vi "Build Profile Header Commands.vi"(8 "error in":errorcluster, 9 "Profile Name":string, 10 "Profile Number":u32=1 min=1 step=1, 11 "F4T in":refnum<class "F4T.lvclass">) -> (0 "error out":errorcluster, 2 "Profile Header Commands":T1[](array[typedef]), 3 "F4T out":refnum<class "F4T.lvclass">)   [LabVIEW 2018, in "F4T.lvlib" / "F4T.lvclass"]
uses:
  F4T.lvclass
  Custom Controls/Command Data.ctl
  PPLs/Temp Chamber/Parent/Temp Chamber.lvlibp/Temp Chamber.lvclass
  PPLs/Temp Chamber/Parent/Configuration.lvlibp/Configuration.lvclass
  C:/Projects/LabVIEW/PPLs/Temp Chamber/Parent/Temp Chamber.lvlibp/Temp Chamber.lvclass
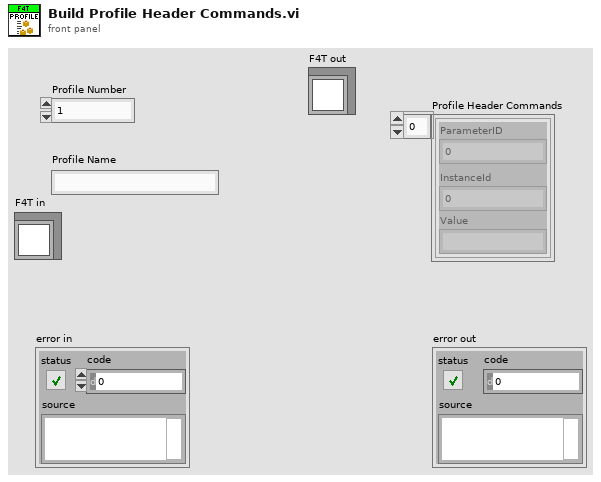
[diagram p1: front panel]
types:
  T1 = typedef "F4T.lvlib/F4T.lvclass/Command Data.ctl" = cluster{"ParameterID":u32, "InstanceId":u32, "Value":string}
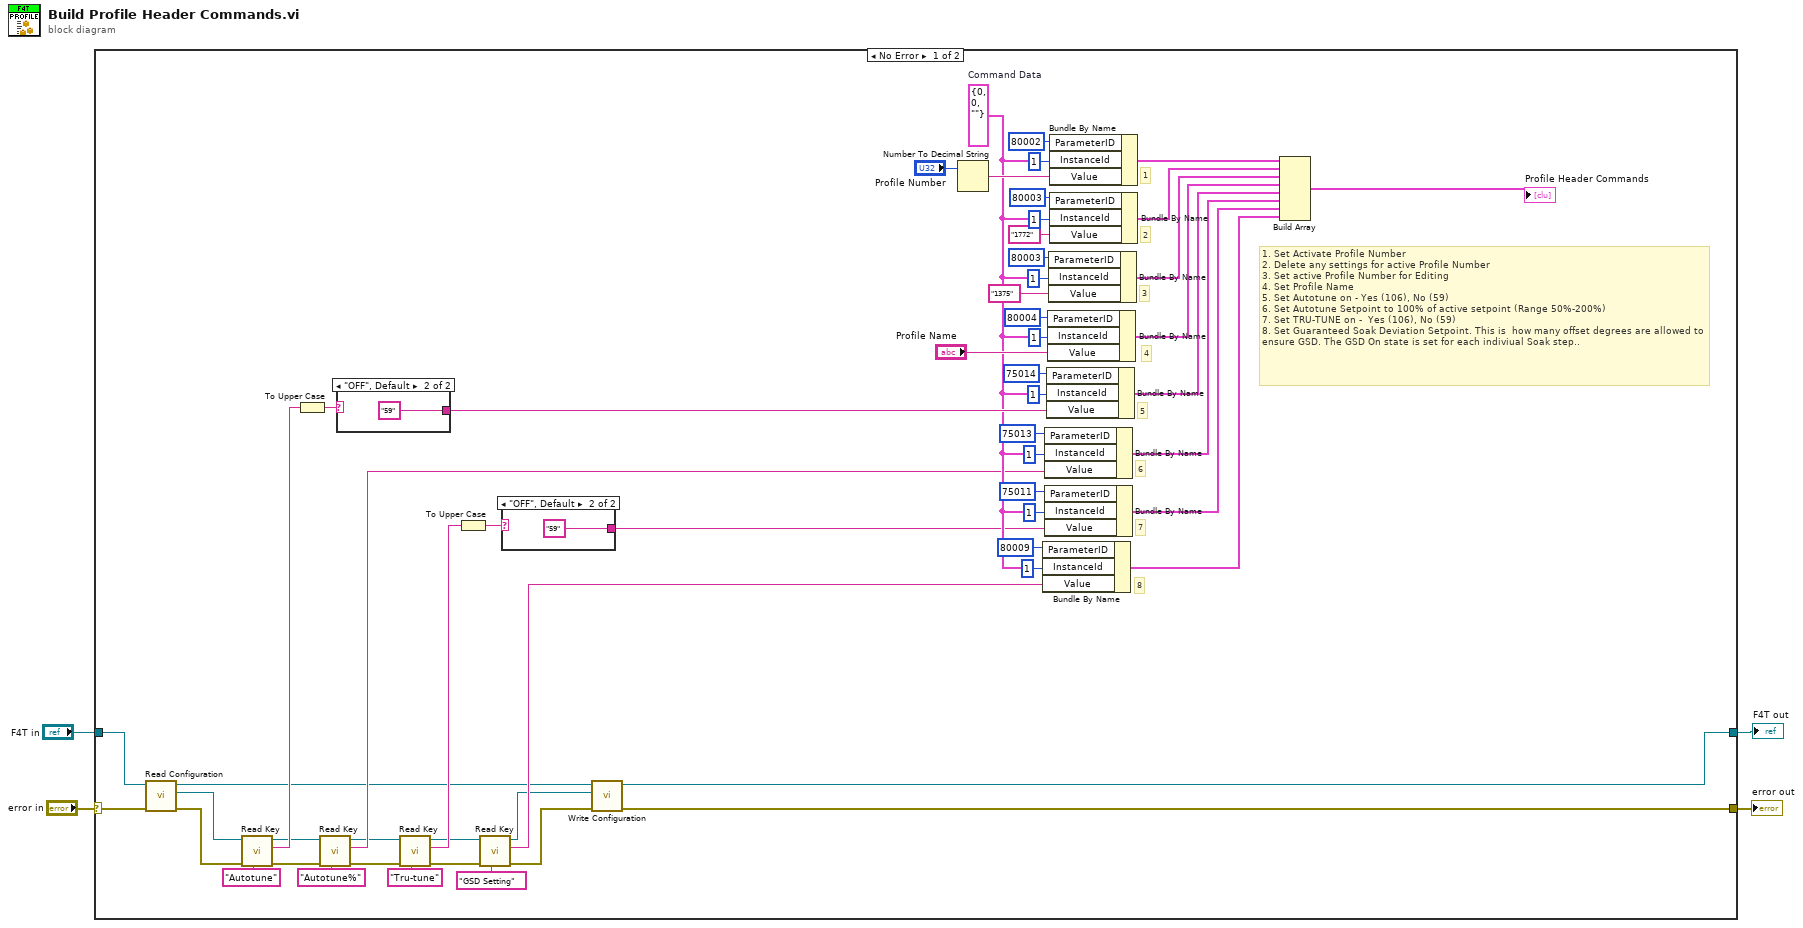
[diagram p0: block diagram]
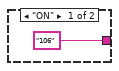
[diagram p2: hidden frame]
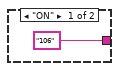
[diagram p3: hidden frame]
diagram:
  n1 = case shown="No Error" "error in" {
    selector: "error in" -> [w29 w68]
    tunnel: [w8 w68] -> w3
    tunnel: "F4T in" -> [w30 w67]
    tunnel: [w7 w67] -> w1
    frame No Error {
      w40 = T1 {"ParameterID"=0, "InstanceId"=0, "Value"=""}  # Command Data
      # "8"
      # "7"
      # "6"
      # "5"
      # "4"
      # "3"
      # "2"
      # "1"
      # "1. Set Activate Profile Number\n2. Delete any settings for active Profile Number\n3. Set active Profile Number for Editing\n4. Set Profile Name \n5. Set Autotune on - Yes (106), No (59)\n6. Set Autotune Setpoint to 100% of active setpoint (Range 50%-200%)\n7. Set TRU-TUNE on -  Yes (106), No (59)\n8. Set Guaranteed Soak Deviation Setpoint. This is  how many offset degrees are allowed to ensure GSD. The GSD On state is set for each indiviual Soak step.."
      n2 = call "Read Configuration.vi"("error in (no error)"=w29, "Temp Chamber in"=w30) -> ("error out"=w28:errorcluster, "Configuration"=w27:refnum<class "Configuration.lvclass">, "Temp Chamber out"=w10:refnum<class "F4T.lvclass">)  [unwired: 7 in]
      n3 = call "Read Key.vi"("Key:"="Autotune", "error in"=w28, "Configuration in"=w27) -> ("error out"=w22:errorcluster, "Value"=w25:string, "Configuration out"=w23:refnum<class "Configuration.lvclass">)  [unwired: 6 in]
      n4 = To Upper Case(1:w25) -> (0:w24:string)
      n5 = call "Read Key.vi"("Key:"="Autotune%", "error in"=w22, "Configuration in"=w23) -> ("error out"=w17:errorcluster, "Value"=w20:string, "Configuration out"=w18:refnum<class "Configuration.lvclass">)  [unwired: 6 in]
      n6 = case shown="\"OFF\", Default" w24 {
        tunnel: ["106" ("Value") "59" ("Value")] -> w47
        frame "ON" {
        }
        frame "OFF", Default {
        }
      }
      n7 = call "Read Key.vi"("Key:"="Tru-tune", "error in"=w17, "Configuration in"=w18) -> ("error out"=w5:errorcluster, "Value"=w16:string, "Configuration out"=w6:refnum<class "Configuration.lvclass">)  [unwired: 6 in]
      n8 = To Upper Case(1:w16) -> (0:w14:string)
      n9 = call "Read Key.vi"("Key:"="GSD Setting", "error in"=w5, "Configuration in"=w6) -> ("error out"=w9:errorcluster, "Value"=w12:string, "Configuration out"=w11:refnum<class "Configuration.lvclass">)  [unwired: 6 in]
      n10 = case shown="\"OFF\", Default" w14 {
        tunnel: ["106" ("Value") "59" ("Value")] -> w15
        frame "ON" {
        }
        frame "OFF", Default {
        }
      }
      n11 = call "Write Configuration.vi"("error in (no error)"=w9, "Configuration"=w11, "Temp Chamber in"=w10) -> ("error out"=w8:errorcluster, "Temp Chamber out"=w7:refnum<class "F4T.lvclass">)  [unwired: 7 in]
      n12 = Number To Decimal String(number="Profile Number") -> (decimal integer string=w61:string)  [unwired: 1 in]
      n13 = Bundle By Name(cluster=w40, "ParameterID"=u32 80009, "InstanceId"=u32 1, "Value"=w12) -> (w32:T1)
      n14 = Bundle By Name(cluster=w40, "ParameterID"=u32 75013, "InstanceId"=u32 1, "Value"=w20) -> (w34:T1)
      n15 = Bundle By Name(cluster=w40, "ParameterID"=u32 75011, "InstanceId"=u32 1, "Value"=w15) -> (w33:T1)
      n16 = Bundle By Name(cluster=w40, "ParameterID"=u32 75014, "InstanceId"=u32 1, "Value"=w47) -> (w35:T1)
      n17 = Bundle By Name(cluster=w40, "ParameterID"=u32 80004, "InstanceId"=u32 1, "Value"="Profile Name") -> (w36:T1)
      n18 = Bundle By Name(cluster=w40, "ParameterID"=u32 80003, "InstanceId"=u32 1, "Value"="1375") -> (w37:T1)
      n19 = Bundle By Name(cluster=w40, "ParameterID"=u32 80002, "InstanceId"=u32 1, "Value"=w61) -> (w39:T1)
      n20 = Bundle By Name(cluster=w40, "ParameterID"=u32 80003, "InstanceId"=u32 1, "Value"="1772") -> (w38:T1)
      n21 = Build Array(w39, w38, w37, w36, w35, w34, w33, w32) -> (→"Profile Header Commands":T1[])
    }
    frame Error {
    }
  }
  "error out" <- w3
  "F4T out" <- w1
